vi "Path2.vi"(8 "error in (no error)":errorcluster caption="错误输入（无错误）") -> (0 "error out":errorcluster caption="错误输出", 3 "拆分的路径":path)   [LabVIEW 2018]
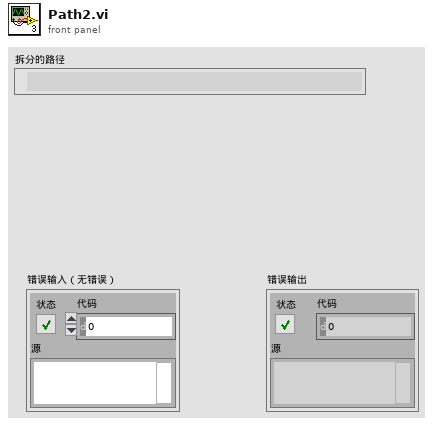
[diagram p1: front panel]
types:
  T1 = enum32{"invalid app kind", "Development System", "Run Time System", "Student Edition", "Embedded LabVIEW", "Evaluation", "Custom"}
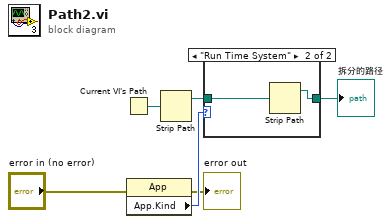
[diagram p0: block diagram]
diagram:
  n1 = Current VI's Path() -> (path=w5:path)
  n2 = property class="App"(error in="error in (no error)") -> (error out=→"error out":errorcluster, "App.Kind"=w6:T1)  [unwired: 1 in, 1 out]
  n3 = Strip Path(path=w5) -> (stripped path=w4:path)  [unwired: 1 out]
  n4 = case shown="\"Run Time System\"" w6 {
    tunnel: w4 -> [w7 w9]
    tunnel: [w7 w8] -> w3
    frame "Development System", Default {
    }
    frame "Run Time System" {
      n5 = Strip Path(path=w9) -> (stripped path=w8:path)  [unwired: 1 out]
    }
  }
  "拆分的路径" <- w3
